vi "Quiescent Current Consumption Test.vi"(0 "TSM context":T1) -> (15 "error out":errorcluster)   [LabVIEW 2020]
doc: "VI determines the current consumption of DUT during no stimulus conditions."
uses:
  <vilib>/NI_TestStand_SemiconductorModule/NI_TestStand_Semiconductor_Module.lvlibp/PinMap/General/SemiconductorModuleContext.ctl
  Common/Instrument Control/DCPower/SSC DCPower/Measure/SSC DCPower Measurement Mode.ctl
  <vilib>/NI_TestStand_SemiconductorModule/NI_TestStand_Semiconductor_Module.lvlibp/PinMap/TagProvider/TSM_Pin.ctl
  Common/Instrument Control/DCPower/SSC DCPower/SSC DCPower Measure.vi
  <vilib>/NI_TestStand_SemiconductorModule/NI_TestStand_Semiconductor_Module.lvlibp/PinMap/General/Publish/PublishDataDoubleFunctionalTest.vi
  <vilib>/NI_TestStand_SemiconductorModule/NI_TestStand_Semiconductor_Module.lvlibp
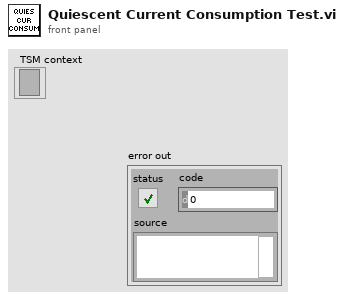
[diagram p1: front panel]
types:
  T1 = typedef "NI_TestStand_Semiconductor_Module.lvlibp/SemiconductorModuleContext.ctl" = refnum<k7>
  T2 = typedef "NI_TestStand_Semiconductor_Module.lvlibp/TSM_Pin.ctl" = tag
  T3 = typedef "SSC DCPower Measurement Mode.ctl" = enum16{"Auto", "Measure Multiple", "Software Triggers"}
  T4 = typedef "TSM SSC DCPower.ctl" = cluster{"Pin Query Context":refnum<class "MultiplePinMultipleSessionQueryContext.lvclass">, "SSC":T5[], "Site Numbers":i32[], "Pins":T6[], "Pins Expanded":T8[]}
  T5 = typedef "SSC DCPower.ctl" = cluster{"Session":refnum<k15>, "Chan":string, "Channel List":string}
  T6 = typedef "TSM Pin Information.ctl" = cluster{"Pin":tag, "Type":T7, "Count":i32}
  T7 = typedef "TSM Pin Type Identifier.ctl" = enum8{"DUT Pin", "System Pin", "Pin Group", "Not Determined"}
  T8 = typedef "TSM Expanded Pin Information.ctl" = cluster{"Pin":tag, "Type":T7, "Index":i32}
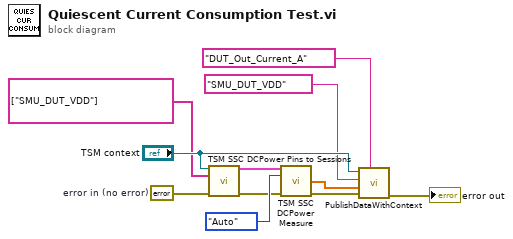
[diagram p0: block diagram]
diagram:
  w10 = errorcluster {"status"=FALSE, "code"=0, "source"=""}  # error in (no error)
  n1 = call "TSM SSC DCPower Pins to Sessions.vi"("TSM context"="TSM context", "Pins"=tag[] ["SMU_DUT_VDD"], "error in"=w10) -> ("DCPower TSM Out"=w6:T4, "error out"=w7:errorcluster)  [unwired: 11 in]
  n2 = call "TSM SSC DCPower Measure.vi"("DCPower TSM in"=w6, "Measurement Mode"=SSC_DCPower_Measurement_Mode."Auto", "error in"=w7) -> ("Current Measurements (A)"=w5:dbl[], "error out"=w2:errorcluster)  [unwired: 9 in, 2 out]
  n3 = call-poly <vilib>:"PublishDataWithContext.vi"("Published Data Id"=tag "DUT_Out_Current_A", "error in (no error)"=w2, "Data In"=w5, "Pin"=T2 "SMU_DUT_VDD", "Semiconductor Module Context"="TSM context") -> ("error out"=→"error out":errorcluster)  [unwired: 5 in, 1 out]
